vi "Generate Measurement.vi"(8 "error in (no error)":errorcluster, 11 "VISA resource name":refnum<visa-resource-name>="GPIB0::8::INSTR") -> (0 "error out":errorcluster)   [LabVIEW 2019, in "DS360.lvlib"]
uses:
  DS360.lvlib
panel:
  in  "stop":bool
  in  "Disable Out":bool
  in  "Enable Out":bool
  in  "Frequency (Hz)":dbl=1000.0
  in  "Amplitude (Vrms)":dbl=5.0
  in  "Serial Configuration":T1={"Baud Rate"=9600, "Parity"=0, "Data Bits"=8, "Stop Bits"=10, "Flow Control"=2} {"Flow Control" items=["None"=0, "RTS/CTS"=2]; "Stop Bits" items=["1.0"=10, "1.5"=15, "2.0"=20]; "Data Bits" items=["7"=7, "8"=8]; "Parity" items=["None", "Odd", "Even", "Mark", "Space"]; "Baud Rate" items=["300"=300, "600"=600, "1200"=1200, "2400"=2400, "4800"=4800, "9600"=9600, "19200"=19200, "38400"=38400, "57600"=57600, "115200"=115200]}
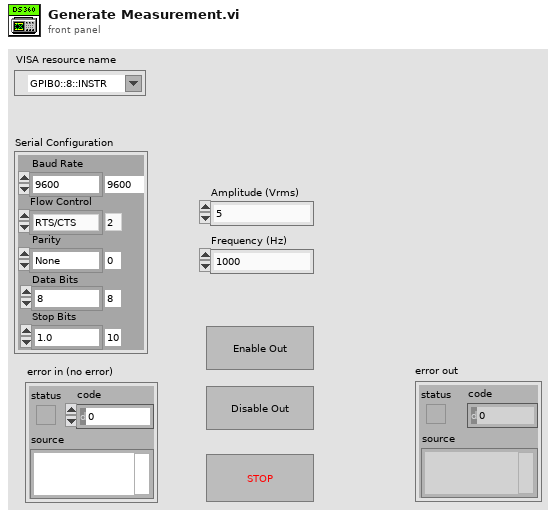
[diagram p1: front panel]
types:
  T1 = cluster{"Baud Rate":u32, "Parity":u16, "Data Bits":u16, "Stop Bits":u16, "Flow Control":u16}
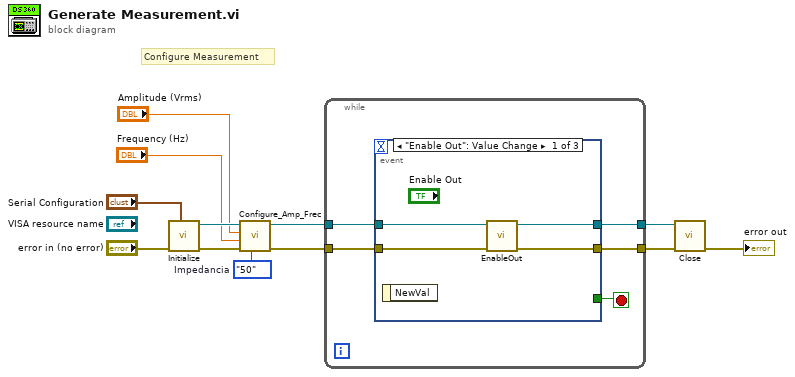
[diagram p0: block diagram]
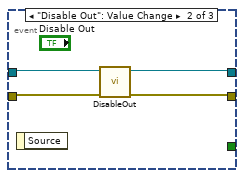
[diagram p2: hidden frame]
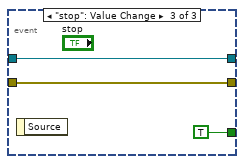
[diagram p3: hidden frame]
diagram:
  w5 = enum16{"50", "600", "HiZ"}."50"  # Impedancia
  # "Configure Measurement"
  n1 = call "Initialize.vi"("Serial Configuration"="Serial Configuration", "error in (no error)"="error in (no error)") -> ("error out"=w11:errorcluster, "VISA resource name out"=w12:refnum<visa-resource-name>)  [unwired: 8 in]
  n2 = call "Configure_Amp_Frec.vi"("Impedancia"=w5, "error in (no error)"=w11, "Frequency (Hz)"="Frequency (Hz)", "Amplitude (Vrms)"="Amplitude (Vrms)", "VISA resource name"=w12) -> ("error out"=w3:errorcluster, "VISA resource name out"=w4:refnum<visa-resource-name>)  [unwired: 5 in]
  n3 = while {
    tunnel: w4 -> [w16]
    tunnel: w3 -> [w15]
    tunnel: [w14] -> w2
    tunnel: [w13] -> w1
    stop <- w17 stop-if-true
    n4 = event shown="[0] \"Enable Out\": Value Change" {
      selector: _ -> [_ _ _]
      dyn-events: _ -> [_ _ _]
      timeout: _ -> [_ _ _]
      tunnel: [_ _ TRUE] -> w17
      tunnel: w16 -> [w21 w24 w27]
      tunnel: w15 -> [w20 w25 w26]
      tunnel: [w19 w22 w27] -> w14
      tunnel: [w18 w23 w26] -> w13
      event "Enable Out": Value Change {
        n5 = event-data() -> ()  [unwired: 1 in, 1 out]
        n6 = call "EnableOut.vi"("error in (no error)"=w20, "VISA resource name"=w21) -> ("error out"=w18:errorcluster, "VISA resource name out"=w19:refnum<visa-resource-name>)  [unwired: 8 in]
      }
      event "Disable Out": Value Change {
        n7 = event-data() -> ()  [unwired: 1 in, 1 out]
        n8 = call "DisableOut.vi"("error in (no error)"=w25, "VISA resource name"=w24) -> ("error out"=w23:errorcluster, "VISA resource name out"=w22:refnum<visa-resource-name>)  [unwired: 8 in]
      }
      event "stop": Value Change {
        n9 = event-data() -> ()  [unwired: 1 in, 1 out]
      }
    }
  }
  n10 = call "Close.vi"("error in (no error)"=w1, "VISA resource name"=w2) -> ("error out"=→"error out":errorcluster)  [unwired: 9 in]
